vi "CAENHV Get Ch Param Prop Info.vi"(7 "ParName":string, 8 "error in (no error)":errorcluster, 9 "Ch":u16, 10 "slot":u16, 11 "handle":i32) -> (0 "error out":errorcluster, 2 "PARAM_TYPE":T2, 3 "PARAM_MODE":T1)   [LabVIEW 2012, in "CAENHVWrapper.lvlib"]
doc: "CAENHVLIB_API CAENHVRESULT CAENHV_GetChParamProp(int handle, \n ushort slot, ushort Ch, const char *ParName, const char *PropName, void *retval);"
uses:
  CAENHVWrapper.lvlib
  Types/PARAM_TYPE.ctl
  Types/PARAM_MODE.ctl
  CAENHVWrapper.dll
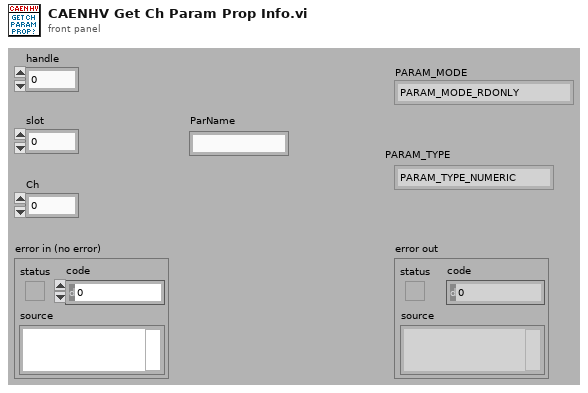
[diagram p1: front panel]
types:
  T1 = typedef "CAENHVWrapper.lvlib/PARAM_MODE.ctl" = enum32{"PARAM_MODE_RDONLY", "PARAM_MODE_WRONLY", "PARAM_MODE_RDWR"}
  T2 = typedef "CAENHVWrapper.lvlib/PARAM_TYPE.ctl" = enum32{"PARAM_TYPE_NUMERIC", "PARAM_TYPE_ONOFF", "PARAM_TYPE_CHSTATUS", "PARAM_TYPE_BDSTATUS", "PARAM_TYPE_BINARY", "PARAM_TYPE_STRING"}
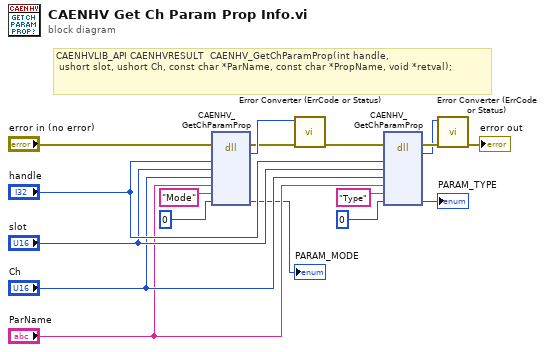
[diagram p0: block diagram]
diagram:
  # "CAENHVLIB_API CAENHVRESULT  CAENHV_GetChParamProp(int handle, \n ushort slot, ushort Ch, const char *ParName, const char *PropName, void *retval);"
  n1 = dll-call lib="CAENHVWrapper.*" fn="CAENHV_GetChParamProp"(error in="error in (no error)", "handle"="handle", "slot"="slot", "Ch"="Ch", "ParName"="ParName", "PropName"="Mode", "retval"=u32 0) -> (error out=w15:errorcluster, "return type"=w16:i32, "retval"=→"PARAM_MODE":u32)  [unwired: 7 in, 1 out]
  n2 = call "Error Converter (ErrCode or Status).vi"("error in (no error)"=w15, "error code"=w16) -> ("error out"=w13:errorcluster)  [unwired: 9 in]
  n3 = dll-call lib="CAENHVWrapper.*" fn="CAENHV_GetChParamProp"(error in=w13, "handle"="handle", "slot"="slot", "Ch"="Ch", "ParName"="ParName", "PropName"="Type", "retval"=u32 0) -> (error out=w11:errorcluster, "return type"=w10:i32, "retval"=→"PARAM_TYPE":u32)  [unwired: 7 in, 1 out]
  n4 = call "Error Converter (ErrCode or Status).vi"("error in (no error)"=w11, "error code"=w10) -> ("error out"=→"error out":errorcluster)  [unwired: 9 in]
